vi "Test Read Raw Data.vi"() -> ()   [LabVIEW 2015, in "KIT QV.lvlib"]
doc: "Read QDEvent log file."
uses:
  KIT QV.lvlib
  <vilib>/Waveform/DWDTOps.llb/DWDT Boolean Array to Digital.vi
panel:
  out "Mixed Signal Graph":T1(graph)
  in  "QDEvent file":path=path "M:/Brand/KIT-QV/QRam33/QDEvent_H11M44S24_D17-M09-Y2015.Log"
  out "text":string
  out "Bit 15 TS":timestamp[](array[timestamp]) format="%^<%H:%M:%S%6u>T"
  out "Bit 14 TS":timestamp[](array[timestamp]) format="%^<%H:%M:%S%6u>T"
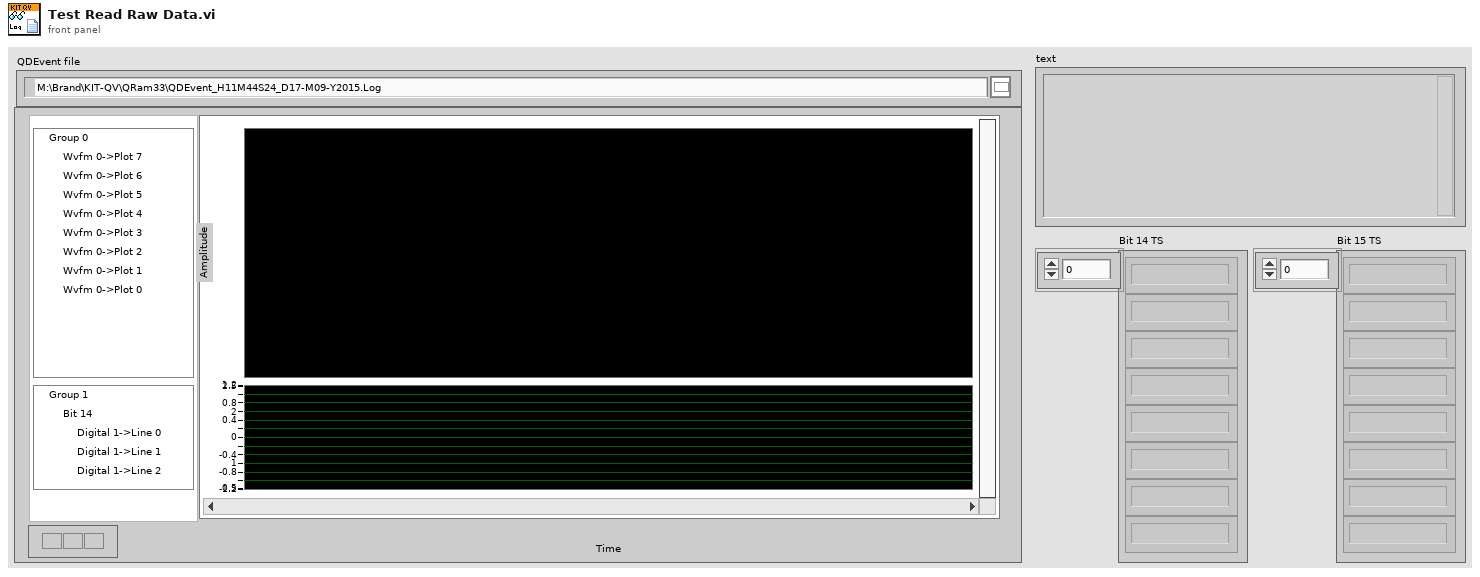
[diagram p1: front panel]
types:
  T1 = cluster{waveform(dbl)[], "digital waveform":digitalwaveform, "digital waveform":digitalwaveform}
  T2 = enum16{"open", "replace", "create", "open or create", "replace or create", "replace or create with confirmation"}
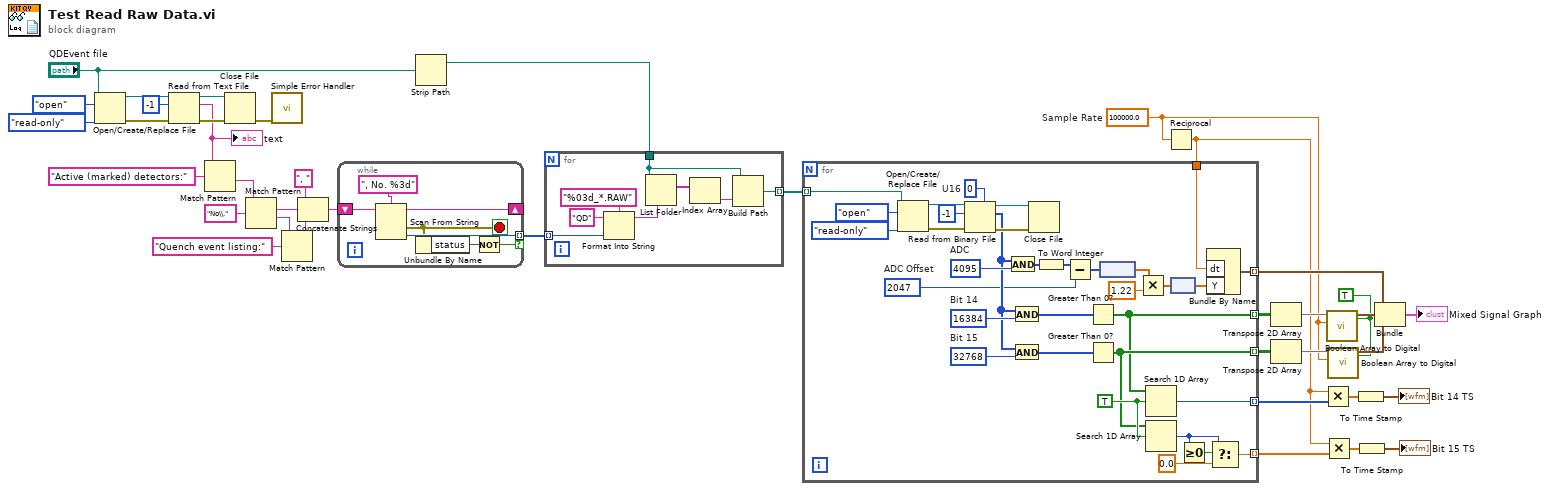
[diagram p0: block diagram]
diagram:
  w10 = TRUE ("compress data (F)")
  w9 = 100000.0  # Sample Rate
  n1 = Open/Create/Replace File(file path (use dialog)="QDEvent file", operation (0:open)=T2."open", access (0:read/write)=enum16{"read/write", "read-only", "write-only"}."read-only") -> (refnum out=w37:refnum<file>, error out=w36:errorcluster)  [unwired: 3 in, 1 out]
  n2 = Read from Text File(file (use dialog)=w37, count=-1, error in=w36) -> (refnum out=w34:refnum<file>, text=w31:string, error out=w35:errorcluster)  [unwired: 1 in, 1 out]
  "text" <- w31
  n3 = Match Pattern(string=w31, regular expression="Active (marked) detectors:") -> (after substring=w29:string)  [unwired: 1 in, 3 out]
  n4 = Close File(refnum=w34, error in=w35) -> (error out=w32:errorcluster)  [unwired: 1 out]
  n5 = Match Pattern(string=w29, regular expression="No\\.") -> (match substring=w27:string, after substring=w26:string)  [unwired: 1 in, 2 out]
  n6 = call <vilib>:"Simple Error Handler.vi"("error in (no error)"=w32) -> ()  [unwired: 4 in, 5 out]
  n7 = Match Pattern(string=w26, regular expression="Quench event listing:") -> (before substring=w24:string)  [unwired: 1 in, 3 out]
  n8 = Concatenate Strings(", " ("string"), w27, w24) -> (w23:string)
  n9 = while {
    shift-right: [w45] -> _
    shift-left: w23 -> [w46]
    tunnel: [w43] -> w19 mode=indexing if=w41
    stop <- w42 stop-if-true
    n10 = Scan From String(format string=", No. %3d", input string=w46) -> (remaining string=w45:string, error out=w42:errorcluster, output 1=w43:i32)  [unwired: 3 in, 1 out]
    n11 = Unbundle By Name(w42) -> ("status"=w40:bool)
    n12 = Not(x=w40) -> (.not. x?=w41:bool)
  }
  n13 = Strip Path(path="QDEvent file") -> (stripped path=w20:path)  [unwired: 1 out]
  n14 = for {
    tunnel: w20 -> [w50]
    tunnel: w19 -> [w48] mode=indexing
    tunnel: [w47] -> w18 mode=indexing
    n15 = Format Into String(format string="%03d_*.RAW", initial string="QD" ("regular expression"), w48) -> (resulting string=w52:string)  [unwired: 1 in, 1 out]
    n16 = List Folder(path=w50, pattern=w52) -> (filenames=w51:string[])  [unwired: 2 in, 3 out]
    n17 = Index Array(array=w51) -> (element=w49:string)  [unwired: 1 in]
    n18 = Build Path(base path=w50, name or relative path=w49) -> (appended path=w47:path)
  }
  n19 = Reciprocal(x=w9) -> (1/x=w7:dbl)
  n20 = for {
    tunnel: w18 -> [w76] mode=indexing
    tunnel: [w68] -> w11 mode=indexing
    tunnel: [w73] -> w8 mode=indexing
    tunnel: [w59] -> w6 mode=indexing
    tunnel: [w71] -> w17 mode=indexing
    tunnel: [w67] -> w15 mode=indexing
    tunnel: w7 -> [w63]
    w56 = i16 2047  # ADC Offset
    w72 = TRUE
    w79 = u16 32768  # Bit 15
    w81 = u16 16384  # Bit 14
    w82 = u16 4095  # ADC
    w85 = u16 0  # U16
    n21 = Open/Create/Replace File(file path (use dialog)=w76, operation (0:open)=T2."open", access (0:read/write)=enum16{"read/write", "read-only", "write-only"}."read-only") -> (refnum out=w65:refnum<file>, error out=w64:errorcluster)  [unwired: 3 in, 1 out]
    n22 = Read from Binary File(5:w85, 8:w64, 10:-1 ("count (1)"), 11:w65) -> (0:w84:errorcluster, 2:w80:u16[], 3:w83:refnum<file>)  [unwired: 2 in, 1 out]
    n23 = And(x=w80, y=w82) -> (x .and. y?=w58:u16[])
    n24 = And(x=w80, y=w81) -> (x .and. y?=w78:u16[])
    n25 = And(x=w80, y=w79) -> (x .and. y?=w77:u16[])
    n26 = Close File(refnum=w83, error in=w84) -> ()  [unwired: 2 out]
    n27 = To Word Integer(number=w58) -> (16bit integer=w55:i16[])
    n28 = Subtract(x=w55, y=w56) -> (x-y=w57:i16[])
    n29 = Greater Than 0?(x=w78) -> (x > 0?=w67:bool[])
    n30 = Greater Than 0?(x=w77) -> (x > 0?=w71:bool[])
    n31 = node(w57) -> (w74:dbl[unit][])
    n32 = Multiply(x=w74, y=1.22) -> (x*y=w70:dbl[unit][])
    n33 = Search 1D Array(1D array=w67, element=w72) -> (index of element=w73:i32)  [unwired: 1 in]
    n34 = Search 1D Array(1D array=w71, element=w72) -> (index of element=w60:i32)  [unwired: 1 in]
    n35 = node(w70) -> (w69:dbl[])
    n36 = Greater Or Equal To 0?(x=w60) -> (x >= 0?=w62:bool)
    n37 = Bundle By Name("dt"=w63, "Y"=w69) -> (w68:waveform(dbl))  [unwired: 1 in]
    n38 = Select(t=w60, s=w62, f=0.0) -> (s? t:f=w59:dbl)
  }
  n39 = Transpose 2D Array(2D array=w15) -> (transposed array=w14:bool[][])
  n40 = Transpose 2D Array(2D array=w17) -> (transposed array=w16:bool[][])
  n41 = Multiply(x=w7, y=w8) -> (x*y=w5:dbl[])
  n42 = Multiply(x=w7, y=w6) -> (x*y=w4:dbl[])
  n43 = call-poly <vilib>:"Boolean Array to Digital.vi"("compress data (F)"=w10, "sample rate"=w9, "boolean array"=w14) -> ("digital waveform"=w12:digitalwaveform)  [unwired: 7 in, 1 out]
  n44 = call-poly <vilib>:"Boolean Array to Digital.vi"("compress data (F)"=w10, "sample rate"=w9, "boolean array"=w16) -> ("digital waveform"=w13:digitalwaveform)  [unwired: 7 in, 1 out]
  n45 = To Time Stamp(1:w5) -> (0:→"Bit 14 TS":timestamp[])
  n46 = To Time Stamp(1:w4) -> (0:→"Bit 15 TS":timestamp[])
  n47 = Bundle(w11, "digital waveform"=w12, "digital waveform"=w13) -> (→"Mixed Signal Graph":T1)  [unwired: 1 in]
